vi "Tx Cyclic Clear.vi"(8 "error in (no error)":errorcluster, 11 "Tx Cyclic":T1) -> (0 "error out":errorcluster)   [LabVIEW 2020, in "985x Support Addon Engine.lvlib"]
uses:
  985x Support Addon Engine.lvlib
  Types/Cyclic Frame Info.ctl
  Types/Tx Cyclic Session.ctl
  Types/FPGA Refnum.ctl
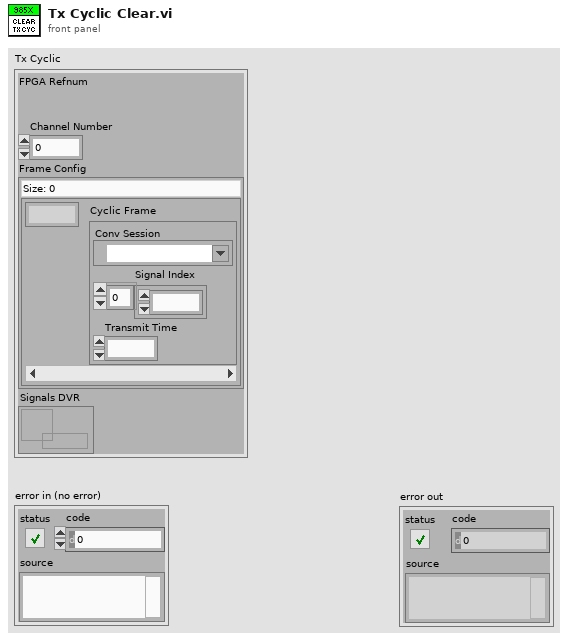
[diagram p1: front panel]
types:
  T1 = typedef "985x Support Addon Engine.lvlib/Tx Cyclic Session.ctl" = cluster{"FPGA Refnum":T2, "Channel Number":u32, "Frame Config":map{u32, T3}, "Signals DVR":refnum<data-value>}
  T2 = typedef "985x Support Addon Engine.lvlib/FPGA Refnum.ctl" = refnum<k20>
  T3 = typedef "985x Support Addon Engine.lvlib/Cyclic Frame Info.ctl" = cluster{"Conv Session":refnum<k21>, "Signal Index":u32[], "Transmit Time":dbl}
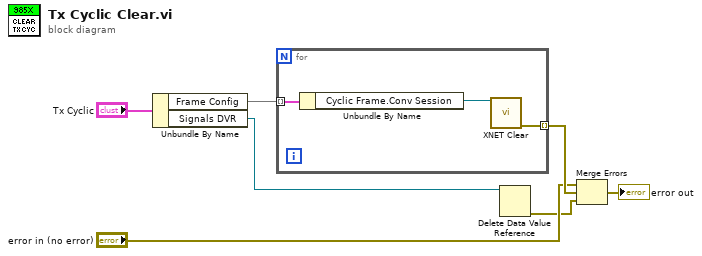
[diagram p0: block diagram]
diagram:
  n1 = Unbundle By Name("Tx Cyclic") -> ("Frame Config"=w6:map{u32, T3}, "Signals DVR"=w5:refnum<data-value>)
  n2 = for {
    tunnel: w6 -> [w10] mode=indexing
    tunnel: [w8] -> w4 mode=indexing
    n3 = Unbundle By Name(w10) -> ("Cyclic Frame.Conv Session"=w9:refnum<k21>)
    n4 = call <vilib>:"XNET Clear.vi"("session in"=w9) -> ("error out"=w8:errorcluster)  [unwired: 14 in]
  }
  n5 = Delete Data Value Reference(data value reference=w5) -> (error out=w2:errorcluster)  [unwired: 1 in, 1 out]
  n6 = Merge Errors("error in (no error)", w4, w2) -> (→"error out":errorcluster)
